vi "Open Gyro.vi"(8 "Gain":dbl=0.07, 9 "Analog Channel":T1=enum."AI 1", 11 "Gyro ID (1 or 2)":i32) -> ()   [LabVIEW 2014]
uses:
  <vilib>/Rock Robotics/SystemInterfaces/AI/FPGA_AIChannel.ctl
  Gyro Global.vi
  Robot Global Data.vi
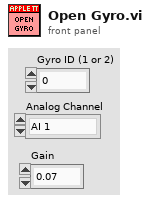
[diagram p1: front panel]
types:
  T1 = typedef "FPGA_AIChannel.ctl" = enum8{"AI 0", "AI 1", "AI 2", "AI 3", "AI MXP 0", "AI MXP 1", "AI MXP 2", "AI MXP 3", "Invalid"}
  T2 = typedef "WPI_AnalogChannelDevRef.ctl" = cluster{"DevStatus":errorcluster, "Controller":T3, "Analog Channel":T1}
  T3 = typedef "FPGA_TypedefAnalogModule.ctl" = enum16{"Controller 1"}
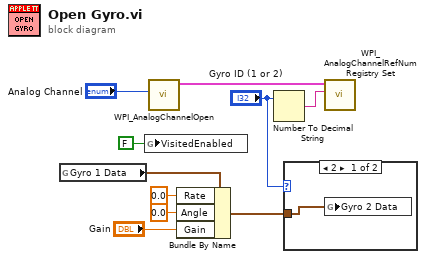
[diagram p0: block diagram]
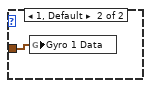
[diagram p2: hidden frame]
diagram:
  n1 = global read "Robot Global Data.vi" "Gyro 1 Data"() -> (w1:cluster{"Rate":dbl, "Angle":dbl, "Gain":dbl})
  n2 = global write "Gyro Global.vi" "VisitedEnabled"(FALSE ("VisitedEnabled")) -> ()
  n3 = call <vilib>:"WPI_AnalogChannelOpen.vi"("Analog Channel"="Analog Channel") -> ("AIDeviceRef"=w9:T2)  [unwired: 9 in, 1 out]
  n4 = Bundle By Name(cluster=w1, "Rate"=0.0, "Angle"=0.0, "Gain"="Gain") -> (w2:cluster{"Rate":dbl, "Angle":dbl, "Gain":dbl})
  n5 = Number To Decimal String(number="Gyro ID (1 or 2)") -> (decimal integer string=w7:string)  [unwired: 1 in]
  n6 = case shown="2" "Gyro ID (1 or 2)" {
    tunnel: w2 -> [w11 w12]
    frame 2 {
      n7 = global write "Robot Global Data.vi" "Gyro 2 Data"(w11) -> ()
    }
    frame 1, Default {
      n8 = global write "Robot Global Data.vi" "Gyro 1 Data"(w12) -> ()
    }
  }
  n9 = call <vilib>:"WPI_AnalogChannelRefNum Registry Set.vi"("refnum name"=w7, "AIDeviceRef"=w9) -> ()  [unwired: 8 in, 2 out]
